vi "sokudo-string.vi"(1 "Input":i32[][](array[numeric])) -> (0 "output":string[][](array[string]))   [LabVIEW 2014]
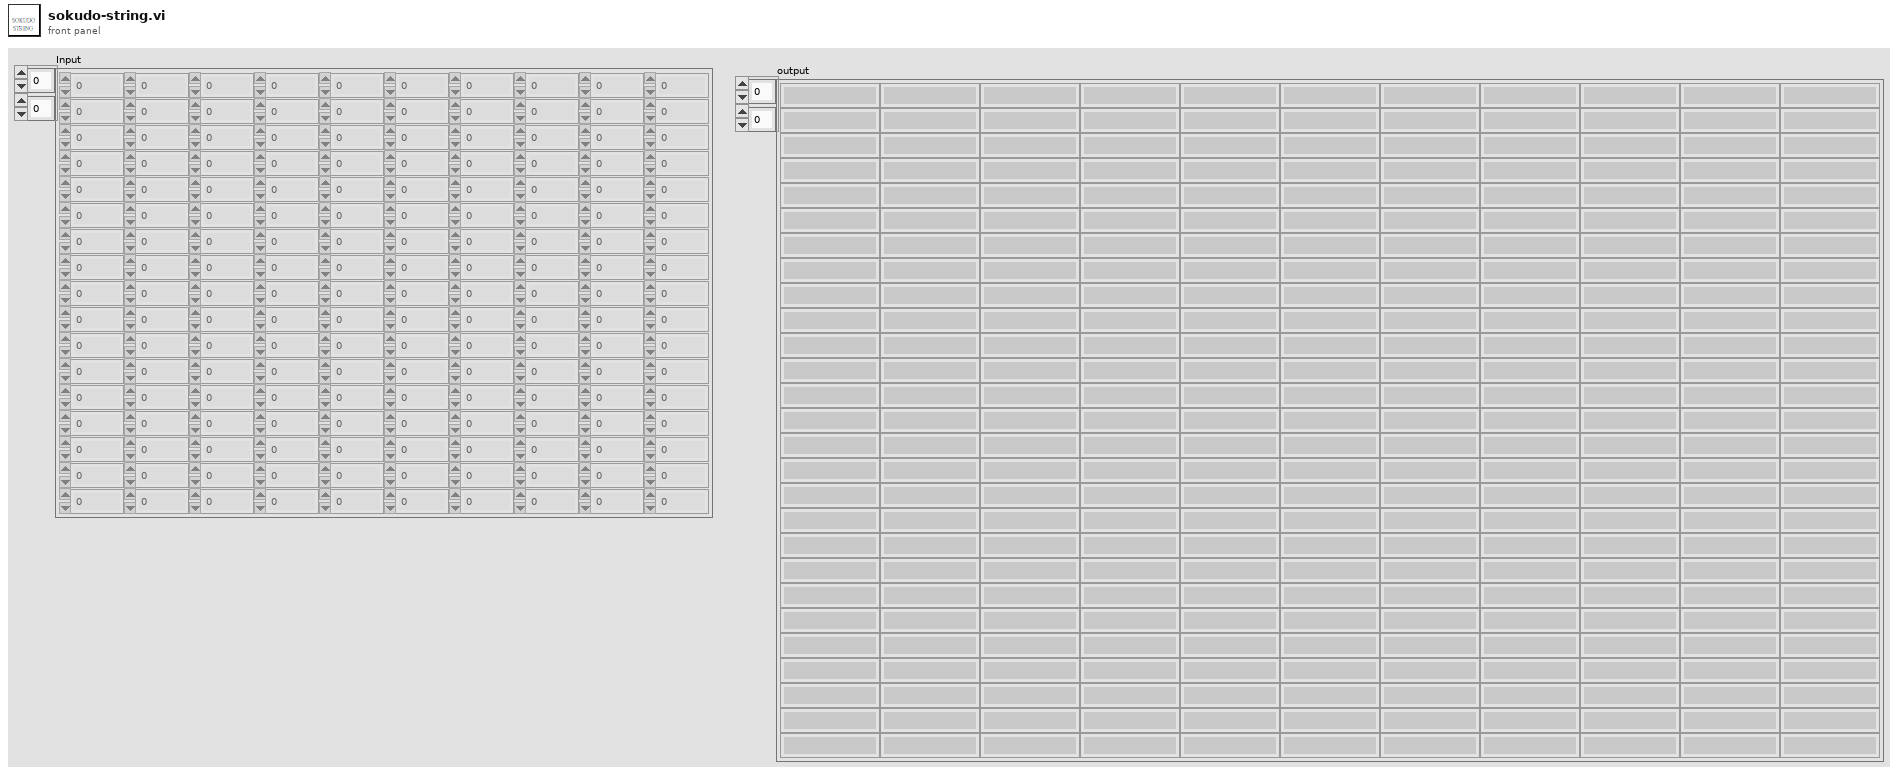
[diagram p1: front panel]
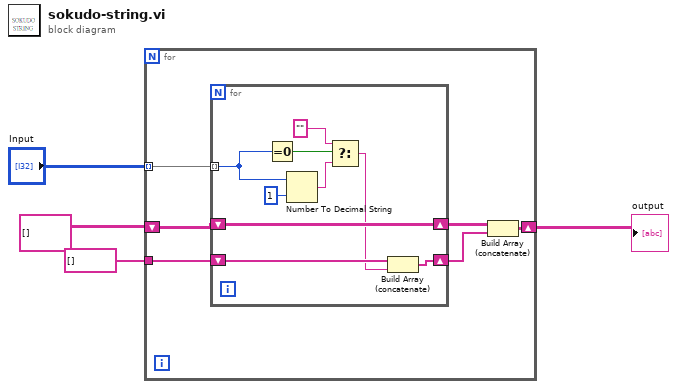
[diagram p0: block diagram]
diagram:
  n1 = for {
    tunnel: "Input" -> [w10] mode=indexing
    shift-right: [w5] -> w2
    shift-left: string[][] [] -> [w9]
    tunnel: string[] [] -> [w7]
    n2 = for {
      tunnel: w10 -> [w17] mode=indexing
      shift-right: [w14] -> w8
      shift-left: w9 -> [w14]
      shift-right: [w11] -> w6
      shift-left: w7 -> [w13]
      n3 = Equal To 0?(x=w17) -> (x = 0?=w19:bool)
      n4 = Number To Decimal String(number=w17, width (-)=i16 1) -> (decimal integer string=w16:string)
      n5 = Select(t="", s=w19, f=w16) -> (s? t:f=w12:string)
      n6 = Build Array (concatenate)(w13, w12) -> (w11:string[])
    }
    n7 = Build Array (concatenate)(w8, w6) -> (w5:string[][])
  }
  "output" <- w2
